vi "Read Sweep Speed (Hz).vi"(8 "error in (no error)":errorcluster, 11 "Laser in":refnum<class "Laser.lvclass">) -> (0 "error out":errorcluster, 2 "Sweep Speed (Hz)":dbl, 3 "Laser out":refnum<class "Laser.lvclass">)   [LabVIEW 2014, in "Laser.lvclass"]
uses:
  Laser.lvclass
  Laser.lvclass/Laser.ctl
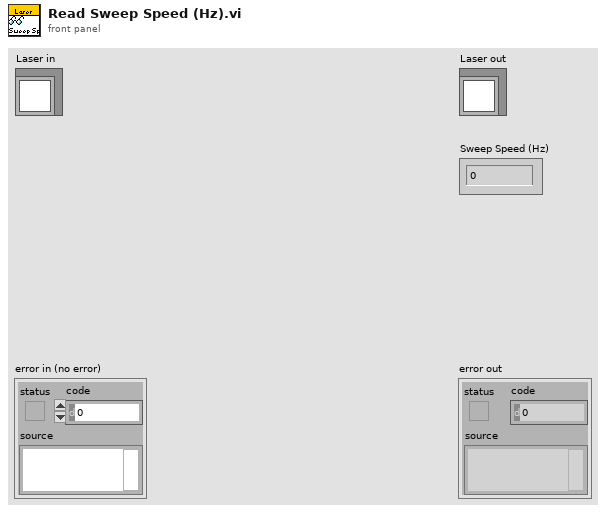
[diagram p1: front panel]
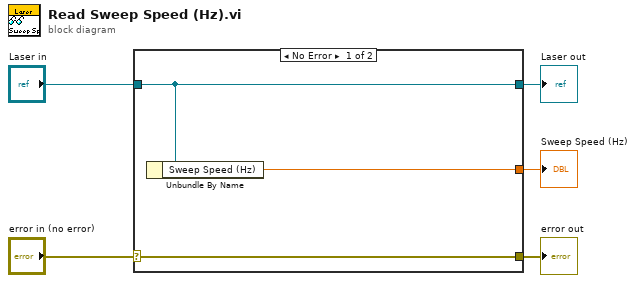
[diagram p0: block diagram]
diagram:
  n1 = case shown="No Error" "error in (no error)" {
    selector: "error in (no error)" -> [w8 w9]
    tunnel: [w8 w9] -> w4
    tunnel: [w7 w10] -> w2
    tunnel: "Laser in" -> [w7 w10]
    tunnel: [w6 _] -> w1
    frame No Error {
      n2 = Unbundle By Name(w7) -> ("Sweep Speed (Hz)"=w6:dbl)
    }
    frame Error {
    }
  }
  "error out" <- w4
  "Laser out" <- w2
  "Sweep Speed (Hz)" <- w1
